vi "Run_Core.vi"(0 "Message Popup in":refnum<class "Assignment Statement.lvclass">, 11 "error in (no error)":errorcluster) -> (4 "Message Popup out":refnum<class "Assignment Statement.lvclass">, 6 "Return":variant, 15 "error out":errorcluster)   [LabVIEW 2016, in "Assignment Statement.lvclass"]
uses:
  Assignment Statement.lvclass
  E:/Repository/LabVIEW Script Language/source code/LSL components/functions/functionsbase/functionbase.lvclass
  Assignment Statement.lvclass/Assignment Statement.ctl
  functionsbase/functionbase.lvclass/functionbase.ctl
  functionsbase/properties/Read Output Terminal.vi
  functionsbase/properties/Read RT Variables.vi
  functionsbase/properties/Read Indent#.vi
  output terminal/Base/Output Terminal.lvclass
  variables/RT Variables/RT Variables.lvclass
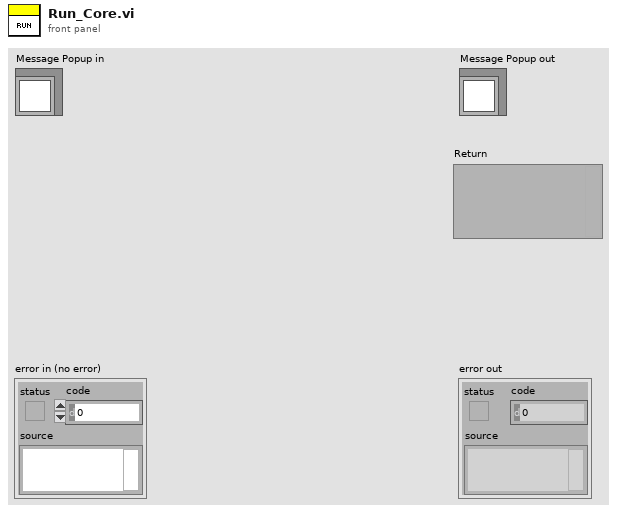
[diagram p1: front panel]
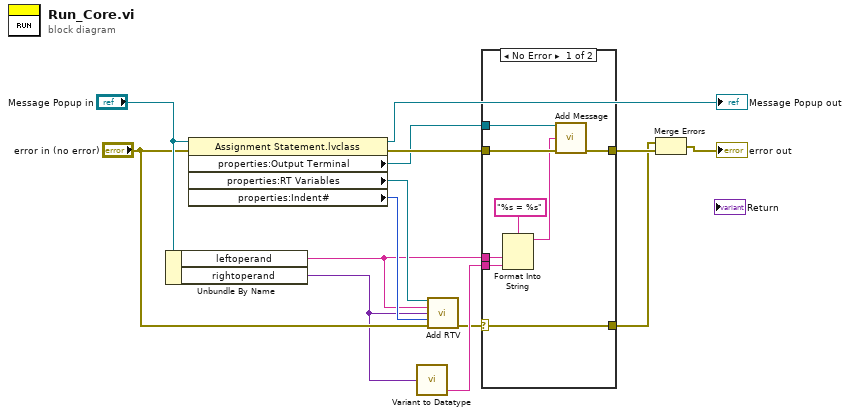
[diagram p0: block diagram]
diagram:
  n1 = Unbundle By Name("Message Popup in") -> ("leftoperand"=w4:string, "rightoperand"=w5:variant)
  n2 = property class="Assignment Statement.lvclass"(reference="Message Popup in", error in="error in (no error)") -> (reference out=→"Message Popup out":refnum<class "Assignment Statement.lvclass">, error out=w8:errorcluster, "properties:Output Terminal"=w6:refnum<class "Output Terminal.lvclass">, "properties:RT Variables"=w9:refnum<class "RT Variables.lvclass">, "properties:Indent#"=w10:i64)
  n3 = call "Variant to Datatype.vi"("Variant"=w5) -> ("Value"=w3:string)  [unwired: 2 in, 2 out]
  n4 = call-dynamic "Add RTV.vi"("RT Variables in"=w9, "RTV name"=w4, "Data"=w5, "Scope"=w10, "error in (no error)"="error in (no error)") -> ("error out"=w2:errorcluster)  [unwired: 9 in, 1 out]
  n5 = case shown="No Error" w2 {
    selector: w2 -> [w15 w24]
    tunnel: w8 -> [w22 w23]
    tunnel: [w21 w23] -> w7
    tunnel: w6 -> [w20 _]
    tunnel: w4 -> [w19 _]
    tunnel: w3 -> [w18 _]
    tunnel: [w15 w24] -> w1
    frame No Error {
      n6 = Format Into String(format string="%s = %s", w19, w18) -> (resulting string=w17:string)  [unwired: 2 in, 1 out]
      n7 = call-dynamic "Add Message.vi"("Output Terminal in"=w20, "Message"=w17, "error in (no error)"=w22) -> ("error out"=w21:errorcluster)  [unwired: 11 in, 1 out]
    }
    frame Error {
    }
  }
  n8 = Merge Errors(w1, w7) -> (→"error out":errorcluster)
